vi "Clear TCP Buffer.vi"(11 "TCP Connection In":refnum<k5>) -> (2 "data out":string, 3 "TCP Connection Out":refnum<k5>)   [LabVIEW 2013, in "TS.lvlib"]
doc: "This VI clears any data in ythe TCP buffer, and throws away any error. It has a zero timeout."
uses:
  TS.lvlib
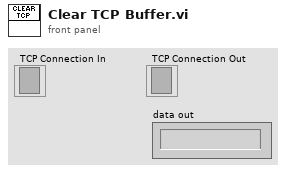
[diagram p1: front panel]
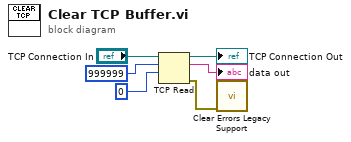
[diagram p0: block diagram]
diagram:
  n1 = TCP Read(connection ID="TCP Connection In", bytes to read=999999, 9:0 ("timeout ms (25000)")) -> (connection ID out=→"TCP Connection Out":refnum<k5>, data out=→"data out":string, error out=w2:errorcluster)  [unwired: 2 in]
  n2 = call "Clear Errors Legacy Support.vi"("error in (no error)"=w2) -> ()  [unwired: 5 in, 2 out]
